vi "New Terminal Visibility Binding.vi"(7 "Initial Visible State (T)":bool=TRUE, 9 "Inverse Binding Logic?":bool, 10 "Control":refnum<vi>) -> (0 "error out":errorcluster, 3 "TerminalVisibilityBinding Out":refnum<class "TerminalVisibilityBinding.lvclass">)   [LabVIEW 2017, in "Transport.lvlib" / "TerminalVisibilityBinding.lvclass"]
doc: "<License>\nCopyright © 2017 Composed Systems, LLC | All rights reserved\nwww.composed.io\n\nAuthor: Ethan Stern <ethan.stern@composed.io>\n\nThis software is provided \"AS IS\" WITHOUT WARRANTIES, either express or implied, AND IS FOR EDUCATIONAL PURPOSES ONLY.\n</License>"
uses:
  TerminalVisibilityBinding.lvclass
  TerminalVisibilityBinding.lvclass/TerminalVisibilityBinding.ctl
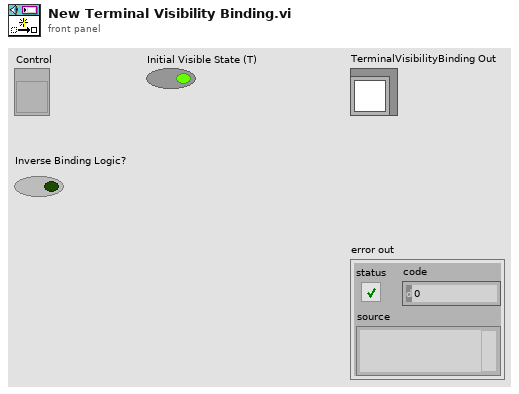
[diagram p1: front panel]
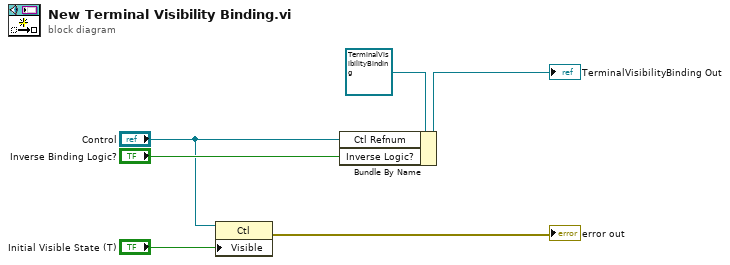
[diagram p0: block diagram]
diagram:
  n1 = property class="Ctl"(reference="Control", "Visible"="Initial Visible State (T)") -> (error out=→"error out":errorcluster)  [unwired: 1 in, 1 out]
  n2 = Bundle By Name(cluster=refnum<class "TerminalVisibilityBinding.lvclass"> refnum ("TerminalReference in"), "Ctl Refnum"="Control", "Inverse Logic?"="Inverse Binding Logic?") -> (→"TerminalVisibilityBinding Out":refnum<class "TerminalVisibilityBinding.lvclass">)
